vi "选择测试项目.vi"() -> (0 "报告测试内容":string, 1 "queue out":refnum<queue>)   [LabVIEW 2015]
panel:
  out "err out":errorcluster caption="err in"
  in  "err in":errorcluster caption="error out"
  out "主状态机状态":T1=enum."等待按键"
  out "项名":T2=["指令测试", "数据测试", "特殊功能测试", "心跳包测试", "升级测试", "中心切换测试", "生成报告"]
  out "选中项目数组":i32[](array[numeric])
  out "选择项目数组":i32[](array[numeric])
  out "总体选择项目":i32[](listbox)
  in  "确认":bool
  in  "全部移除":bool
  in  "全部添加":bool
  in  "移除":bool
  in  "添加":bool
  in  "选中项目":i32[](listbox)
  in  "选择项目":i32[](listbox)
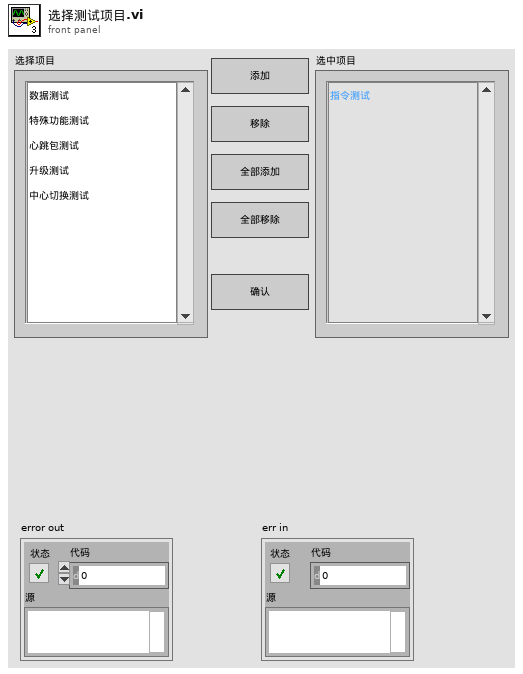
[diagram p1: front panel]
types:
  T1 = typedef "状态机状态.ctl" = enum16{"初始化", "等待按键", "串口操作", "检索模块", "网络测试", "测试项目", "模块参数配置", "指令测试", "数据测试", "特殊功能测试", "心跳包测试", "升级测试", "中心切换测试", "计算测试耗时", "生成报告", "提示消息", "退出"}
  T2 = typedef "测试环节数组.ctl" = string[]
  T3 = typedef "测试状态机.ctl" = enum16{"初始化", "等待按键", "添加", "移除", "全部添加", "全部移除", "显示", "退出"}
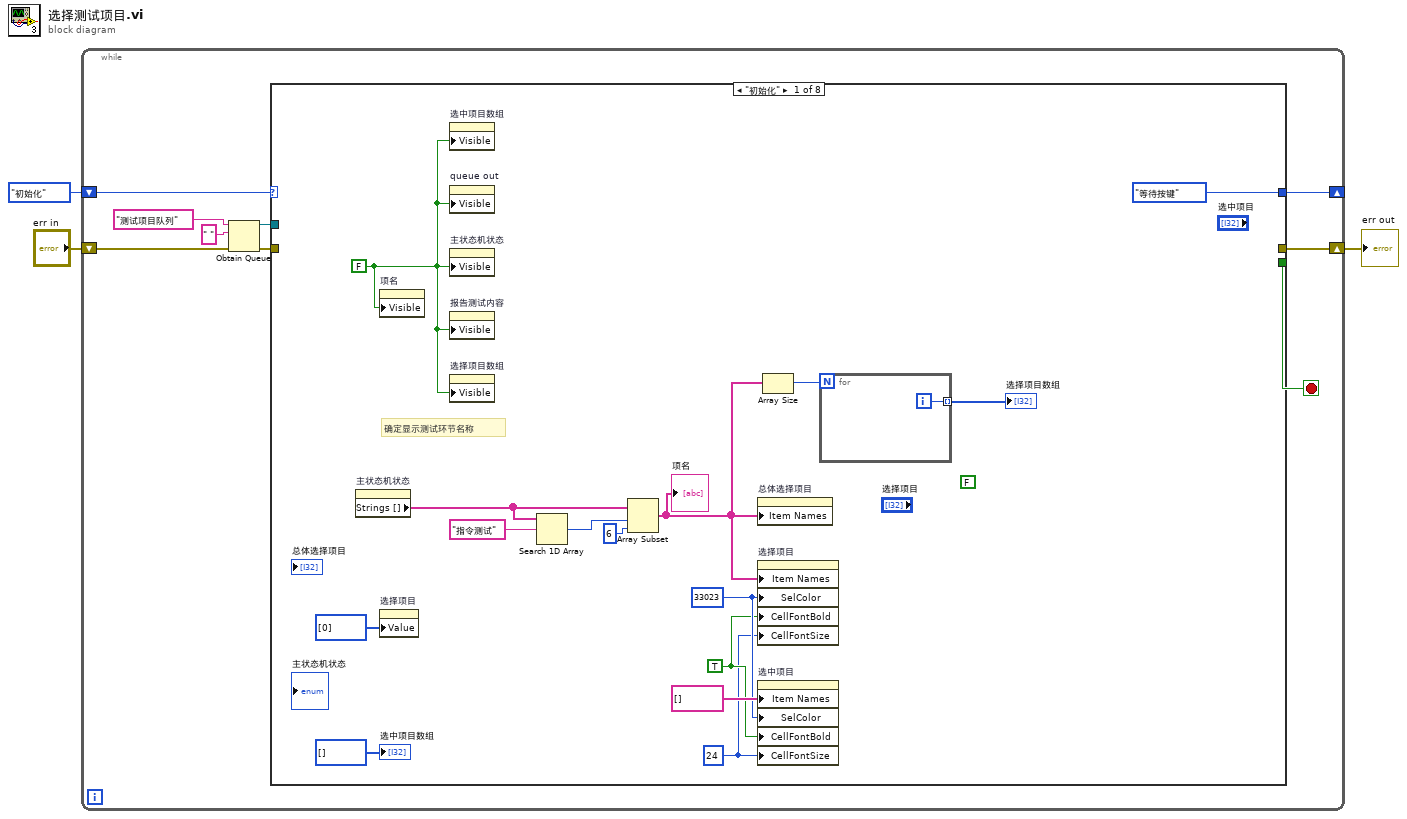
[diagram p0: block diagram]
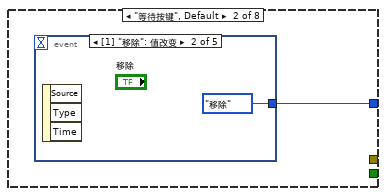
[diagram p2: hidden frame]
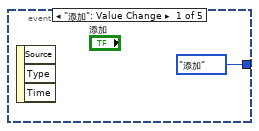
[diagram p3: hidden frame]
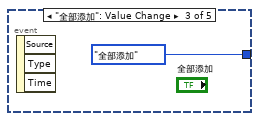
[diagram p4: hidden frame]
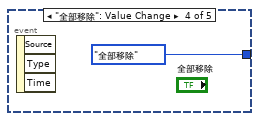
[diagram p5: hidden frame]
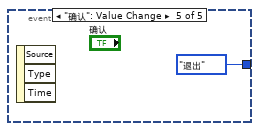
[diagram p6: hidden frame]
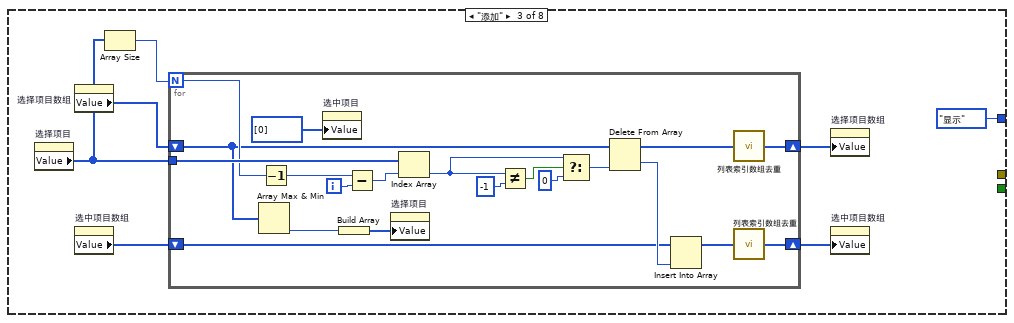
[diagram p7: hidden frame]
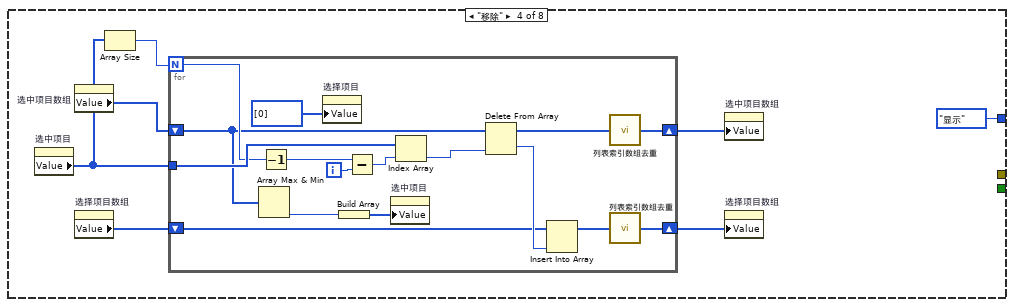
[diagram p8: hidden frame]
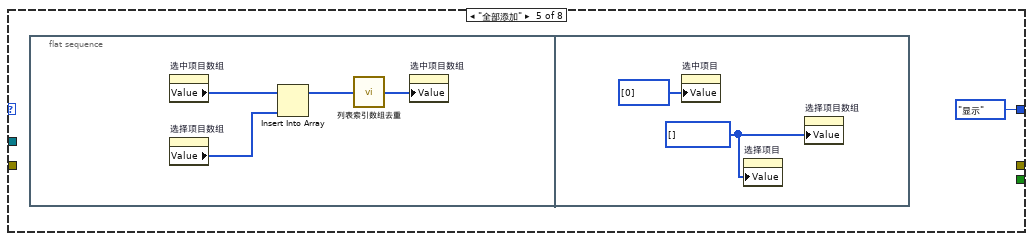
[diagram p9: hidden frame]
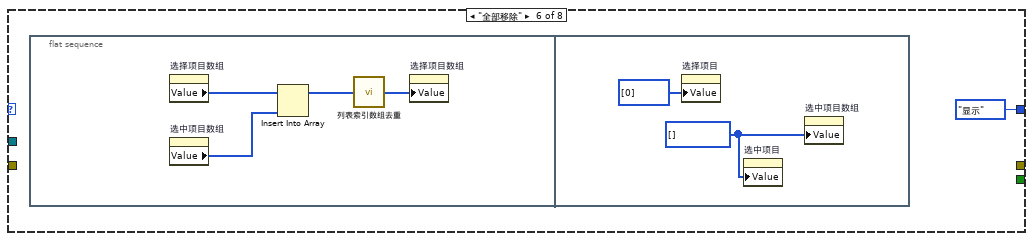
[diagram p10: hidden frame]
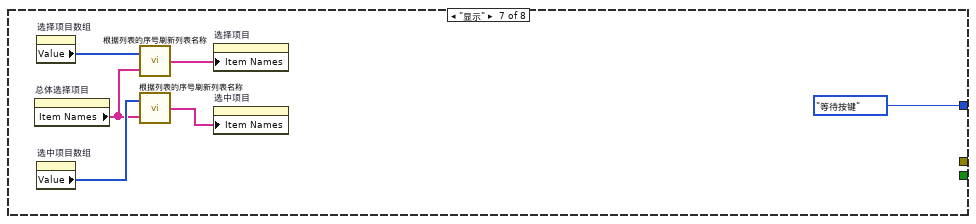
[diagram p11: hidden frame]
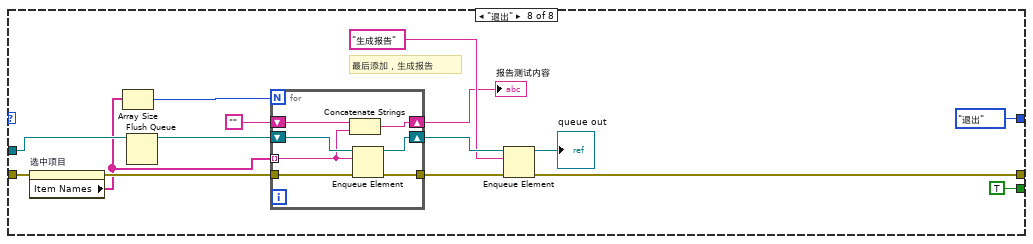
[diagram p12: hidden frame]
diagram:
  n1 = while {
    shift-right: [w10] -> _
    shift-left: 测试状态机."初始化" -> [w12]
    shift-right: [w4] -> w1
    shift-left: "err in" -> [w7]
    stop <- w11 stop-if-true
    n2 = Obtain Queue(name (unnamed)="测试项目队列" ("名称（未命名）"), element data type=" ", error in (no error)=w7) -> (queue out=w6:refnum<queue>, error out=w5:errorcluster)  [unwired: 2 in, 1 out]
    n3 = case shown="\"初始化\"" w12 {
      tunnel: [_ _ _ _ _ _ _ TRUE] -> w11
      tunnel: [测试状态机."等待按键" w29 测试状态机."显示" 测试状态机."显示" 测试状态机."显示" 测试状态机."显示" 测试状态机."等待按键" 测试状态机."退出"] -> w10
      tunnel: w5 -> [_ _ _ _ _ _ _ w116]
      tunnel: w6 -> [_ _ _ _ _ _ _ w114]
      tunnel: [_ _ _ _ _ _ _ w110] -> w4
      frame "初始化" {
        w21 = u32 24 ("活动行:单元格字体:字号")
        w22 = TRUE ("活动行:单元格字体:粗体")
        w23 = u32 33023 ("选择颜色")
        w13 = FALSE ("可见")
        (unwired) FALSE ("可见")
        # "确定显示测试环节名称"
        n4 = property on="主状态机状态" class="Enum (严格)"() -> ("Strings []"=w15:string[])  [unwired: 2 in, 2 out]
        n5 = property on="项名" class="Arr (严格)"("Visible"=w13) -> ()  [unwired: 2 in, 2 out]
        n6 = property on="选择项目" class="LstBox (严格)"("Value"=i32[] [0] ("选择项目")) -> ()  [unwired: 2 in, 2 out]
        n7 = property on="选中项目数组" class="Arr (严格)"("Visible"=w13) -> ()  [unwired: 2 in, 2 out]
        n8 = property on="queue out" class="TypRef (严格)"("Visible"=w13) -> ()  [unwired: 2 in, 2 out]
        n9 = property on="主状态机状态" class="Enum (严格)"("Visible"=w13) -> ()  [unwired: 2 in, 2 out]
        n10 = property on="报告测试内容" class="Str"("Visible"=w13) -> ()  [unwired: 2 in, 2 out]
        n11 = property on="选择项目数组" class="Arr (严格)"("Visible"=w13) -> ()  [unwired: 2 in, 2 out]
        n12 = Search 1D Array(1D array=w15, element="指令测试" ("查找对象")) -> (index of element=w14:i32)  [unwired: 1 in]
        n13 = Array Subset(array=w15, index=w14, length=6 ("长度")) -> (w18:string[])
        "项名" <- w18
        n14 = property on="总体选择项目" class="LstBox (严格)"("Item Names"=w18) -> ()  [unwired: 2 in, 2 out]
        n15 = property on="选择项目" class="LstBox (严格)"("Item Names"=w18, "SelColor"=w23, "CellFontBold"=w22, "CellFontSize"=w21) -> ()  [unwired: 2 in, 2 out]
        n16 = property on="选中项目" class="LstBox (严格)"("Item Names"=string[] [] ("项名"), "SelColor"=w23, "CellFontBold"=w22, "CellFontSize"=w21) -> ()  [unwired: 2 in, 2 out]
        n17 = Array Size(array=w18) -> (size(s)=w25:i32)
        n18 = for {
          N: w25 -> [_]
          tunnel: [w28] -> w26 mode=indexing
          i -> [w28]
        }
        "选择项目数组" <- w26
        "选中项目数组" <- i32[] [] ("选中项目数组")
      }
      frame "等待按键", Default {
        n19 = event shown="[1] \"移除\": 值改变" {
          selector: _ -> [_ _ _ _ _]
          dyn-events: _ -> [_ _ _ _ _]
          timeout: _ -> [_ _ _ _ _]
          tunnel: [测试状态机."添加" 测试状态机."移除" 测试状态机."全部添加" 测试状态机."全部移除" 测试状态机."退出"] -> w29
          event "添加": Value Change {
            n20 = event-data() -> ()  [unwired: 1 in, 3 out]
          }
          event "移除": Value Change {
            n21 = event-data() -> ()  [unwired: 1 in, 3 out]
          }
          event "全部添加": Value Change {
            n22 = event-data() -> ()  [unwired: 1 in, 3 out]
          }
          event "全部移除": Value Change {
            n23 = event-data() -> ()  [unwired: 1 in, 3 out]
          }
          event "确认": Value Change {
            n24 = event-data() -> ()  [unwired: 1 in, 3 out]
          }
        }
      }
      frame "添加" {
        n25 = property on="选择项目" class="LstBox (严格)"() -> ("Value"=w40:i32[])  [unwired: 2 in, 2 out]
        n26 = property on="选择项目数组" class="Arr (严格)"() -> ("Value"=w38:i32[])  [unwired: 2 in, 2 out]
        n27 = property on="选中项目数组" class="Arr (严格)"() -> ("Value"=w35:i32[])  [unwired: 2 in, 2 out]
        n28 = Array Size(array=w40) -> (size(s)=w39:i32)
        n29 = for {
          N: w39 -> [w59]
          tunnel: w40 -> [w61]
          shift-right: [w53] -> w37
          shift-left: w38 -> [w50]
          shift-right: [w52] -> w36
          shift-left: w35 -> [w51]
          i -> [w57]
          n30 = Array Max & Min(array=w50) -> (min index (indices)=w49:i32)  [unwired: 3 out]
          n31 = Decrement(x=w59) -> (x-1=w56:i32)
          n32 = property on="选中项目" class="LstBox (严格)"("Value"=i32[] [0] ("选中项目")) -> ()  [unwired: 2 in, 2 out]
          n33 = Build Array(w49) -> (w48:i32[])
          n34 = Subtract(x=w56, y=w57) -> (x-y=w58:i32)
          n35 = property on="选择项目" class="LstBox (严格)"("Value"=w48) -> ()  [unwired: 2 in, 2 out]
          n36 = Index Array(array=w61, index=w58) -> (element=w43:i32)
          n37 = Not Equal?(x=w43, y=-1) -> (x != y?=w45:bool)
          n38 = Select(t=w43, s=w45, f=0) -> (s? t:f=w44:i32)
          n39 = Delete From Array(array=w50, index=w44) -> (deleted portion=w60:i32, array with subset deleted=w55:i32[])  [unwired: 1 in]
          n40 = Insert Into Array(array=w51, new element=w60) -> (w54:i32[])  [unwired: 1 in]
          n41 = call "列表索引数组去重.vi"("待去重数组"=w55) -> ("数组输出"=w53:i32[])
          n42 = call "列表索引数组去重.vi"("待去重数组"=w54) -> ("数组输出"=w52:i32[])
        }
        n43 = property on="选择项目数组" class="Arr (严格)"("Value"=w37) -> ()  [unwired: 2 in, 2 out]
        n44 = property on="选中项目数组" class="Arr (严格)"("Value"=w36) -> ()  [unwired: 2 in, 2 out]
      }
      frame "移除" {
        n45 = property on="选中项目" class="LstBox (严格)"() -> ("Value"=w62:i32[])  [unwired: 2 in, 2 out]
        n46 = property on="选中项目数组" class="Arr (严格)"() -> ("Value"=w66:i32[])  [unwired: 2 in, 2 out]
        n47 = property on="选择项目数组" class="Arr (严格)"() -> ("Value"=w65:i32[])  [unwired: 2 in, 2 out]
        n48 = Array Size(array=w62) -> (size(s)=w67:i32)
        n49 = for {
          N: w67 -> [w82]
          tunnel: w62 -> [w84]
          shift-right: [w76] -> w64
          shift-left: w66 -> [w73]
          shift-right: [w75] -> w63
          shift-left: w65 -> [w74]
          i -> [w80]
          n50 = Array Max & Min(array=w73) -> (min index (indices)=w72:i32)  [unwired: 3 out]
          n51 = Decrement(x=w82) -> (x-1=w79:i32)
          n52 = property on="选择项目" class="LstBox (严格)"("Value"=i32[] [0] ("选中项目")) -> ()  [unwired: 2 in, 2 out]
          n53 = Build Array(w72) -> (w71:i32[])
          n54 = Subtract(x=w79, y=w80) -> (x-y=w81:i32)
          n55 = property on="选中项目" class="LstBox (严格)"("Value"=w71) -> ()  [unwired: 2 in, 2 out]
          n56 = Index Array(array=w84, index=w81) -> (element=w70:i32)
          n57 = Delete From Array(array=w73, index=w70) -> (deleted portion=w83:i32, array with subset deleted=w78:i32[])  [unwired: 1 in]
          n58 = Insert Into Array(array=w74, new element=w83) -> (w77:i32[])  [unwired: 1 in]
          n59 = call "列表索引数组去重.vi"("待去重数组"=w78) -> ("数组输出"=w76:i32[])
          n60 = call "列表索引数组去重.vi"("待去重数组"=w77) -> ("数组输出"=w75:i32[])
        }
        n61 = property on="选中项目数组" class="Arr (严格)"("Value"=w64) -> ()  [unwired: 2 in, 2 out]
        n62 = property on="选择项目数组" class="Arr (严格)"("Value"=w63) -> ()  [unwired: 2 in, 2 out]
      }
      frame "全部添加" {
        n63 = flat-sequence {
          frame #0 {
            n64 = property on="选中项目数组" class="Arr (严格)"() -> ("Value"=w89:i32[])  [unwired: 2 in, 2 out]
            n65 = property on="选择项目数组" class="Arr (严格)"() -> ("Value"=w88:i32[])  [unwired: 2 in, 2 out]
            n66 = Insert Into Array(array=w89, new element=w88) -> (w87:i32[])  [unwired: 1 in]
            n67 = call "列表索引数组去重.vi"("待去重数组"=w87) -> ("数组输出"=w86:i32[])
            n68 = property on="选中项目数组" class="Arr (严格)"("Value"=w86) -> ()  [unwired: 2 in, 2 out]
          }
          frame #1 {
            w91 = i32[] [] ("选择项目数组")
            n69 = property on="选中项目" class="LstBox (严格)"("Value"=i32[] [0] ("选中项目")) -> ()  [unwired: 2 in, 2 out]
            n70 = property on="选择项目" class="LstBox (严格)"("Value"=w91) -> ()  [unwired: 2 in, 2 out]
            n71 = property on="选择项目数组" class="Arr (严格)"("Value"=w91) -> ()  [unwired: 2 in, 2 out]
          }
        }
      }
      frame "全部移除" {
        n72 = flat-sequence {
          frame #0 {
            n73 = property on="选择项目数组" class="Arr (严格)"() -> ("Value"=w94:i32[])  [unwired: 2 in, 2 out]
            n74 = property on="选中项目数组" class="Arr (严格)"() -> ("Value"=w93:i32[])  [unwired: 2 in, 2 out]
            n75 = Insert Into Array(array=w94, new element=w93) -> (w96:i32[])  [unwired: 1 in]
            n76 = call "列表索引数组去重.vi"("待去重数组"=w96) -> ("数组输出"=w95:i32[])
            n77 = property on="选择项目数组" class="Arr (严格)"("Value"=w95) -> ()  [unwired: 2 in, 2 out]
          }
          frame #1 {
            w97 = i32[] [] ("选择项目数组")
            n78 = property on="选择项目" class="LstBox (严格)"("Value"=i32[] [0] ("选中项目")) -> ()  [unwired: 2 in, 2 out]
            n79 = property on="选中项目" class="LstBox (严格)"("Value"=w97) -> ()  [unwired: 2 in, 2 out]
            n80 = property on="选中项目数组" class="Arr (严格)"("Value"=w97) -> ()  [unwired: 2 in, 2 out]
          }
        }
      }
      frame "显示" {
        n81 = property on="总体选择项目" class="LstBox (严格)"() -> ("Item Names"=w102:string[])  [unwired: 2 in, 2 out]
        n82 = property on="选择项目数组" class="Arr (严格)"() -> ("Value"=w104:i32[])  [unwired: 2 in, 2 out]
        n83 = property on="选中项目数组" class="Arr (严格)"() -> ("Value"=w103:i32[])  [unwired: 2 in, 2 out]
        n84 = call "根据列表的序号刷新列表名称.vi"("总体列表名称数组输入"=w102, "列表序号"=w104) -> ("列表名称数组输出"=w99:string[])
        n85 = call "根据列表的序号刷新列表名称.vi"("总体列表名称数组输入"=w102, "列表序号"=w103) -> ("列表名称数组输出"=w100:string[])
        n86 = property on="选择项目" class="LstBox (严格)"("Item Names"=w99) -> ()  [unwired: 2 in, 2 out]
        n87 = property on="选中项目" class="LstBox (严格)"("Item Names"=w100) -> ()  [unwired: 2 in, 2 out]
      }
      frame "退出" {
        # "最后添加，生成报告"
        n88 = property on="选中项目" class="LstBox (严格)"(error in=w116) -> (error out=w115:errorcluster, "Item Names"=w107:string[])  [unwired: 1 in, 1 out]
        n89 = Array Size(array=w107) -> (size(s)=w117:i32)
        n90 = Flush Queue(queue=w114) -> (queue out=w113:refnum<queue>)  [unwired: 1 in, 2 out]
        n91 = for {
          N: w117 -> [_]
          tunnel: w107 -> [w121] mode=indexing
          shift-right: [w125] -> w112
          shift-left: w113 -> [w126]
          tunnel: w115 -> [w124]
          tunnel: [w123] -> w109
          shift-right: [w122] -> w105
          shift-left: "" -> [w120]
          n92 = Concatenate Strings(w120, w121) -> (w122:string)
          n93 = Enqueue Element(queue=w126, element=w121, error in (no error)=w124) -> (queue out=w125:refnum<queue>, error out=w123:errorcluster)  [unwired: 1 in, 1 out]
        }
        "报告测试内容" <- w105
        n94 = Enqueue Element(queue=w112, element="生成报告" ("名称（未命名）"), error in (no error)=w109) -> (queue out=→"queue out":refnum<queue>, error out=w110:errorcluster)  [unwired: 1 in, 1 out]
      }
    }
  }
  "err out" <- w1
